vi "Conveyor and Shoot Logging.vi"   [LabVIEW 2016]
uses:
  Conveyor and Shoot Logging Values.vi
  Robot Global Data.vi
types:
  T1 = typedef "WPI_DriverStationRobotMode2.ctl" = enum16{"Autonomous Disabled", "Autonomous Enabled", "Teleop Disabled", "Teleop Enabled", "Disconnected", "Finish", "Test Disabled", "Test Enabled", "Emergency Stopped"}
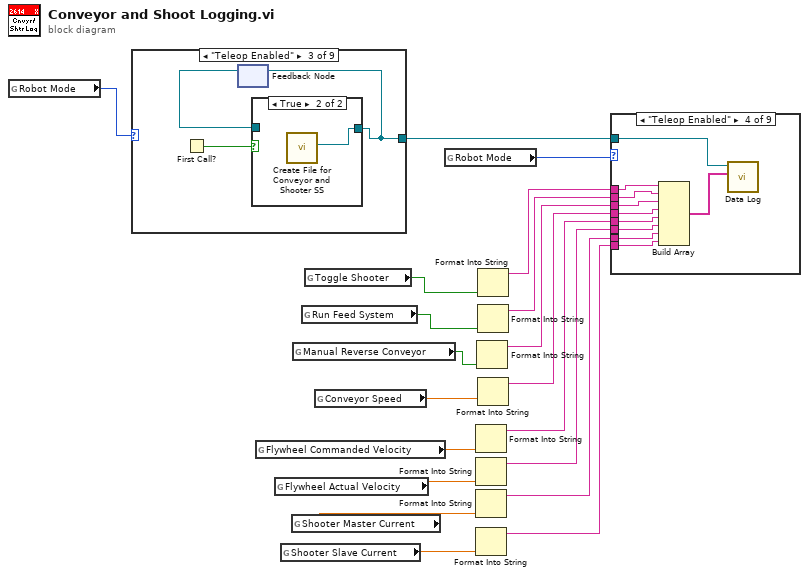
[diagram p0: block diagram]
diagram:
  n1 = global read "Robot Global Data.vi" "Robot Mode"() -> (w14:T1)
  n2 = case shown="\"Teleop Enabled\"" w14 {
    tunnel: [_ _ w20 _ _ _ _ _ _] -> w13
    frame "Autonomous Enabled" {
    }
    frame "Teleop Disabled", Default {
    }
    frame "Teleop Enabled" {
      n3 = First Call?() -> (First Call?: T/F=w22:bool)
      n4 = feedback #1() -> (w21:refnum<file>)  [unwired: 1 in]
      n5 = case shown="True" w22 {
        tunnel: [w23 w24] -> w20
        tunnel: w21 -> [w23 _]
        frame False {
        }
        frame True {
          n6 = call "Create File for Conveyor and Shooter SS.vi"() -> ("File Reference Out"=w24:refnum<file>)  [unwired: 11 in]
        }
      }
      n7 = feedback-in #1(w20) -> ()
    }
    frame "Disconnected" {
    }
    frame "Finish" {
    }
    frame "Test Disabled" {
    }
    frame "Test Enabled" {
    }
    frame "Emergency Stopped" {
    }
    frame "Autonomous Disabled" {
    }
  }
  n8 = global read "Conveyor and Shoot Logging Values.vi" "Flywheel Commanded Velocity"() -> (w4:dbl)
  n9 = global read "Conveyor and Shoot Logging Values.vi" "Flywheel Actual Velocity"() -> (w3:dbl)
  n10 = global read "Conveyor and Shoot Logging Values.vi" "Shooter Slave Current"() -> (w1:dbl)
  n11 = global read "Conveyor and Shoot Logging Values.vi" "Shooter Master Current"() -> (w2:dbl)
  n12 = global read "Conveyor and Shoot Logging Values.vi" "Manual Reverse Conveyor"() -> (w6:bool)
  n13 = global read "Conveyor and Shoot Logging Values.vi" "Run Feed System"() -> (w7:bool)
  n14 = global read "Conveyor and Shoot Logging Values.vi" "Toggle Shooter"() -> (w8:bool)
  n15 = global read "Conveyor and Shoot Logging Values.vi" "Conveyor Speed"() -> (w5:dbl)
  n16 = global read "Robot Global Data.vi" "Robot Mode"() -> (w12:T1)
  n17 = Format Into String(w4) -> (resulting string=w15:string)  [unwired: 3 in, 1 out]
  n18 = Format Into String(w3) -> (resulting string=w11:string)  [unwired: 3 in, 1 out]
  n19 = Format Into String(w2) -> (resulting string=w10:string)  [unwired: 3 in, 1 out]
  n20 = Format Into String(w1) -> (resulting string=w9:string)  [unwired: 3 in, 1 out]
  n21 = Format Into String(w6) -> (resulting string=w17:string)  [unwired: 3 in, 1 out]
  n22 = Format Into String(w8) -> (resulting string=w19:string)  [unwired: 3 in, 1 out]
  n23 = Format Into String(w7) -> (resulting string=w18:string)  [unwired: 3 in, 1 out]
  n24 = Format Into String(w5) -> (resulting string=w16:string)  [unwired: 3 in, 1 out]
  n25 = case shown="\"Teleop Enabled\"" w12 {
    tunnel: w19 -> [_ _ _ w32 _ _ _ _ _]
    tunnel: w18 -> [_ _ _ w31 _ _ _ _ _]
    tunnel: w17 -> [_ _ _ w30 _ _ _ _ _]
    tunnel: w16 -> [_ _ _ w29 _ _ _ _ _]
    tunnel: w15 -> [_ _ _ w28 _ _ _ _ _]
    tunnel: w13 -> [_ _ _ w33 _ _ _ _ _]
    tunnel: w11 -> [_ _ _ w27 _ _ _ _ _]
    tunnel: w10 -> [_ _ _ w26 _ _ _ _ _]
    tunnel: w9 -> [_ _ _ w25 _ _ _ _ _]
    frame "Autonomous Disabled", Default {
    }
    frame "Autonomous Enabled" {
    }
    frame "Teleop Disabled" {
    }
    frame "Teleop Enabled" {
      n26 = Build Array(w32, w31, w30, w29, w28, w27, w26, w25) -> (w34:string[])
      n27 = call "Data Log.vi"("Data In"=w34, "File Reference In"=w33) -> ()  [unwired: 9 in, 1 out]
    }
    frame "Disconnected" {
    }
    frame "Finish" {
    }
    frame "Test Disabled" {
    }
    frame "Test Enabled" {
    }
    frame "Emergency Stopped" {
    }
  }
